vi "delete_collection.vi"(0 "vector_weviate in":refnum<class "vector_weviate.lvclass">, 5 "collection_name":string, 11 "error in (no error)":errorcluster) -> (4 "vector_weviate out":refnum<class "vector_weviate.lvclass">, 15 "error out":errorcluster)   [LabVIEW 2020, in "vector_weviate.lvclass"]
doc: "Deletes the specified collection from the vector store"
uses:
  vector_weviate.lvclass
  vector_weviate.lvclass/vector_weviate.ctl
  <vilib>/httpClient/LabVIEWHTTPClient.lvlib
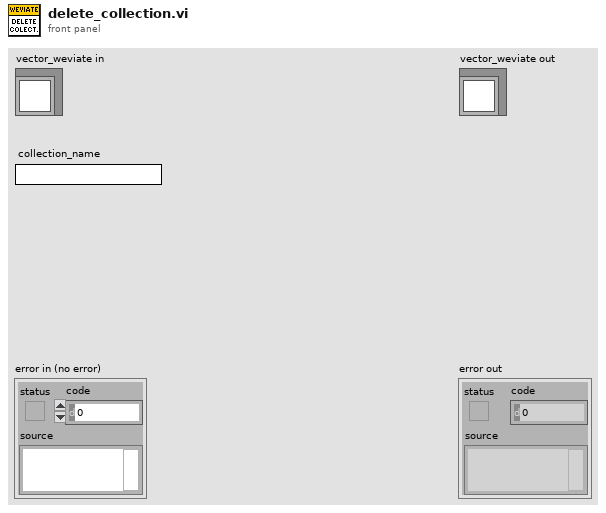
[diagram p1: front panel]
types:
  T1 = typedef "LabVIEWHTTPClient.lvlib/ClientHandle.ctl" = refnum<k1>
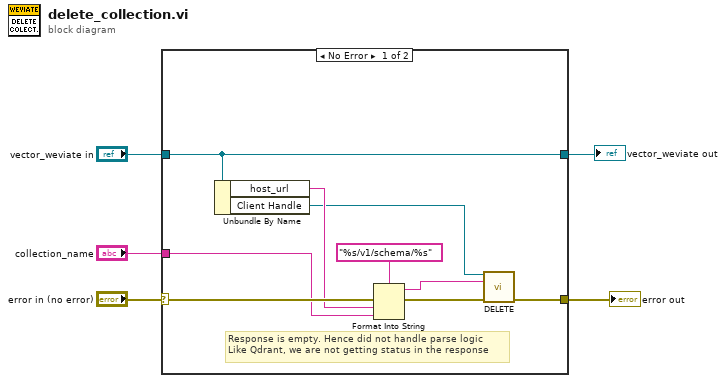
[diagram p0: block diagram]
diagram:
  n1 = case shown="No Error" "error in (no error)" {
    selector: "error in (no error)" -> [w14 w15]
    tunnel: "vector_weviate in" -> [w7 w16]
    tunnel: "collection_name" -> [w11 _]
    tunnel: [w7 w16] -> w2
    tunnel: [w6 w15] -> w1
    frame No Error {
      # "Response is empty. Hence did not handle parse logic\nLike Qdrant, we are not getting status in the response"
      n2 = Unbundle By Name(w7) -> ("host_url"=w13:string, "Client Handle"=w9:T1)
      n3 = Format Into String(format string="%s/v1/schema/%s", error in=w14, w13, w11) -> (resulting string=w8:string, error out=w10:errorcluster)  [unwired: 1 in]
      n4 = call <vilib>:"DELETE.vi"("client handle"=w9, "url"=w8, "error in (no error)"=w10) -> ("error out"=w6:errorcluster)  [unwired: 9 in, 3 out]
    }
    frame Error {
    }
  }
  "error out" <- w1
  "vector_weviate out" <- w2
